vi "Calculate IP Header Checksum.vi"(11 "Payload (bytes)":u8[](array[numeric]) format="%x") -> (3 "checksum":u16 format="%.0x")   [LabVIEW 2021, in "Networking_CIF_U.lvlib"]
uses:
  Networking_CIF_U.lvlib
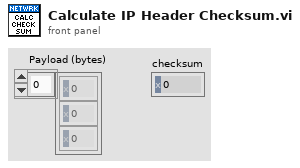
[diagram p1: front panel]
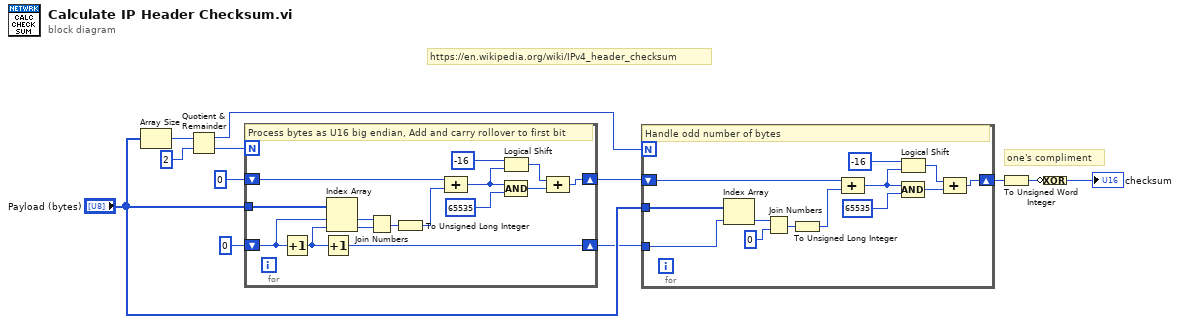
[diagram p0: block diagram]
diagram:
  # "https://en.wikipedia.org/wiki/IPv4_header_checksum"
  # "one's compliment"
  n1 = Array Size(array="Payload (bytes)") -> (size(s)=w12:i32)
  n2 = Quotient & Remainder(x=w12, y=2) -> (x-y*floor(x/y)=w7:i32, floor(x/y)=w10:i32)
  n3 = for {
    N: w10 -> [_]
    tunnel: "Payload (bytes)" -> [w27]
    shift-right: [w24] -> w4
    shift-left: 0 ("index") -> [w26]
    shift-right: [w13] -> w5
    shift-left: u32 0 ("(hi.lo)") -> [w21]
    # "Process bytes as U16 big endian, Add and carry rollover to first bit"
    n4 = Increment(x=w26) -> (x+1=w25:i32)
    n5 = Increment(x=w25) -> (x+1=w24:i32)
    n6 = Index Array(array=w27, index #1=w26, index #2=w25) -> (element #1=w23:u8, element #2=w22:u8)
    n7 = Join Numbers(hi=w23, lo=w22) -> ((hi.lo)=w20:u16)
    n8 = To Unsigned Long Integer(number=w20) -> (unsigned 32bit integer=w19:u32)
    n9 = Compound Arithmetic op=ADD(w21, w19) -> (w17:u32)
    n10 = Logical Shift(y=i16 -16, x=w17) -> (x << y=w15:u32)
    n11 = Compound Arithmetic op=AND(w17, u32 65535 ("value")) -> (w14:u32)
    n12 = Compound Arithmetic op=ADD(w15, w14) -> (w13:u32)
  }
  n13 = for {
    N: w7 -> [_]
    tunnel: "Payload (bytes)" -> [w40]
    shift-right: [w29] -> w3
    shift-left: w5 -> [w37]
    tunnel: w4 -> [w39]
    # "Handle odd number of bytes"
    n14 = Index Array(array=w40, index=w39) -> (element=w38:u8)
    n15 = Join Numbers(hi=w38, lo=u8 0) -> ((hi.lo)=w36:u16)
    n16 = To Unsigned Long Integer(number=w36) -> (unsigned 32bit integer=w35:u32)
    n17 = Compound Arithmetic op=ADD(w37, w35) -> (w33:u32)
    n18 = Logical Shift(y=i16 -16, x=w33) -> (x << y=w31:u32)
    n19 = Compound Arithmetic op=AND(w33, u32 65535 ("value")) -> (w30:u32)
    n20 = Compound Arithmetic op=ADD(w31, w30) -> (w29:u32)
  }
  n21 = To Unsigned Word Integer(number=w3) -> (unsigned 16bit integer=w2:u16)
  n22 = Compound Arithmetic op=XOR(invert w2) -> (→"checksum":u16)
